vi "User Log In (popup).vi"(8 "error in (no error)":errorcluster, 11 "Path":path=path "R:/Freelancing/BEL/RMU LV Code_ver8.0/Data/credentials.txt") -> (0 "error out":errorcluster, 1 "selected account name":string, 2 "test sequence file name":string, 3 "Stop App?":bool, 5 "Name indicator":string caption="Name(min 4 chars)")   [LabVIEW 2021]
uses:
  controls/encryption.ctl
  <vilib>/event_ctls.llb/eventvkey.ctl
  <vilib>/Utility/file.llb/Write Delimited Spreadsheet (string).vi
  <vilib>/Utility/file.llb/Read Delimited Spreadsheet (string).vi
  <vilib>/regexp/Match Regular Expression.xnode
panel:
  in  "test sequence file":u16(ring) caption="Enum" items=["test sequence.seq", "test sequence1.seq", "vishal.seq"]
  out "Tab Control":enum32{"Login account", "Change Password"}(tab)
  in  "Account":enum16{"Administrator", "Operator"}(ring)
  in  "Password":string
  in  "Log In":bool
  out "Attempt":dbl
  out "Attempt (Max)":dbl
  out "lock/unlock":enum32{"lock", "unlock"}(tab)
  in  "Change Password":bool
  in  "Name":string caption="Name(min 4 chars)"
  in  "Account 2":enum16{"Administrator", "Operator"}(ring) caption="Account"
  in  "Password 2":string caption="Password"
  in  "New Password":string
  in  "Confirm Password":string
  in  "Update":bool
  in  "Home":bool
  out "selected account":enum16{"Administrator", "Operator"}(ring)
  # "Please select the appropriate user \naccount, enter the associated \npassword, then select Log In"
  # "Log In attempt"
  # "of"
  # "Please select the appropriate user \naccount, enter the new \npassword, then select Update"
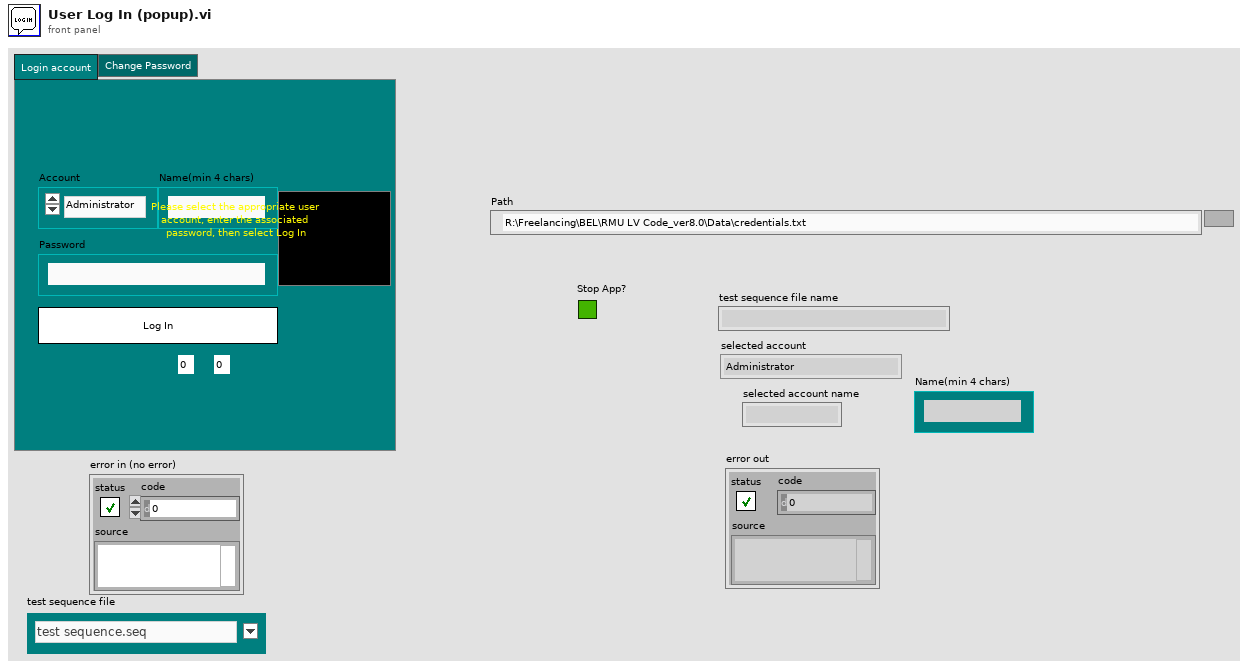
[diagram p1: front panel]
types:
  T1 = typedef "encryption.ctl" = enum16{"encode", "decode"}
  T2 = typedef "eventvkey.ctl" = enum16{"ASCII", "Enter", "Return", "Shift", "Ctrl", "Alt", "Cmd", "Opt", "Caps", "NumLock", "Clear", "Break", "Up", "Down", "Left", "Right", "Insert", "Delete", "Home", "End", "PageUp", "PageDown", "Escape", "Help", "Pause", "ScrollLock", "F1", "F2", "F3", "F4", "F5", "F6", "F7", "F8", "F9", "F10", "F11", "F12", "F13", "F14", "F15", "F16", "F17", "F18", "F19", "F20", "F21", "F22", "F23", "F24", "Play", "VolumeUp", "VolumeDown", "Mute", "Two Byte Char"}
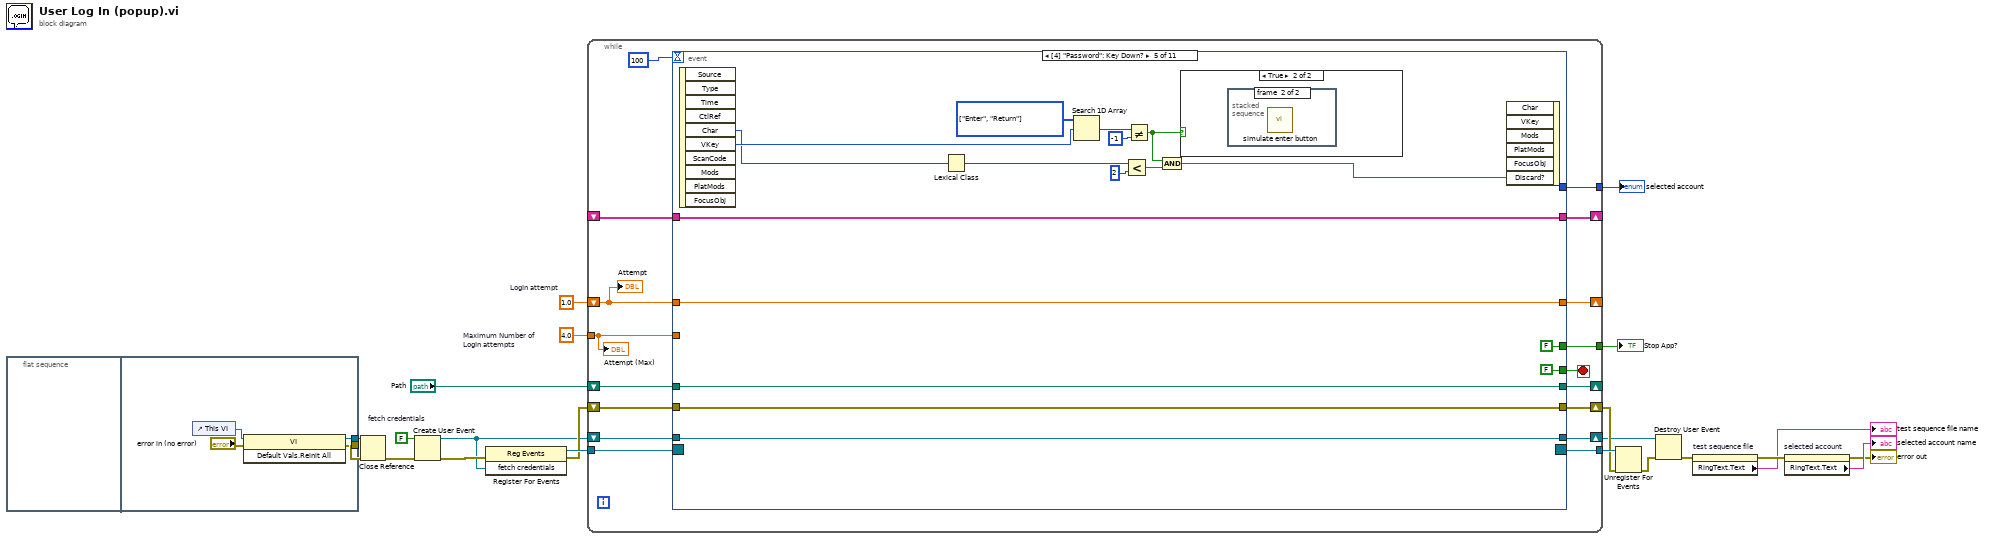
[diagram p0: block diagram]
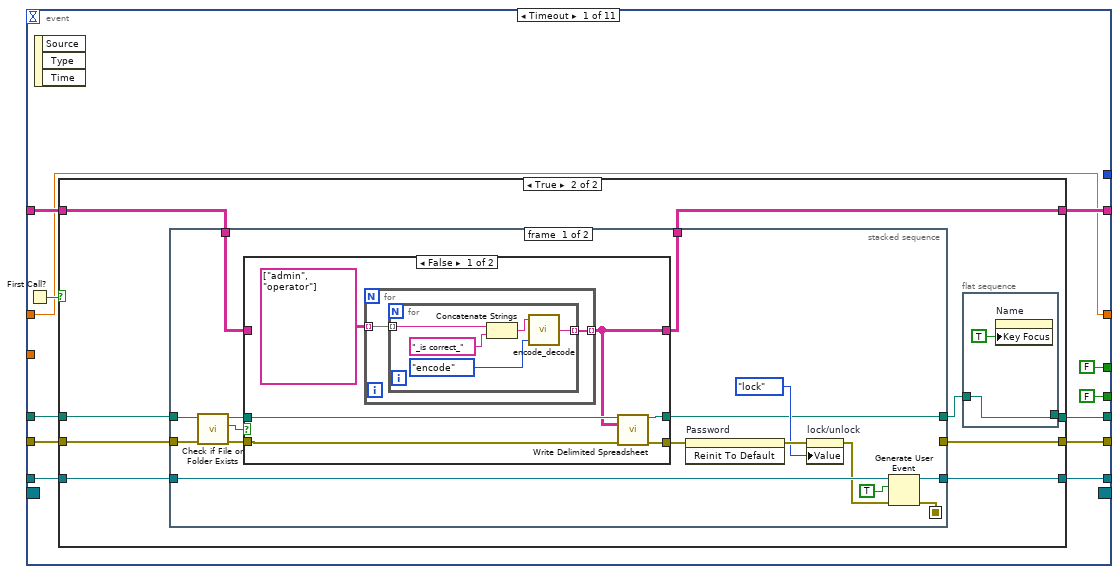
[diagram p2: hidden frame]
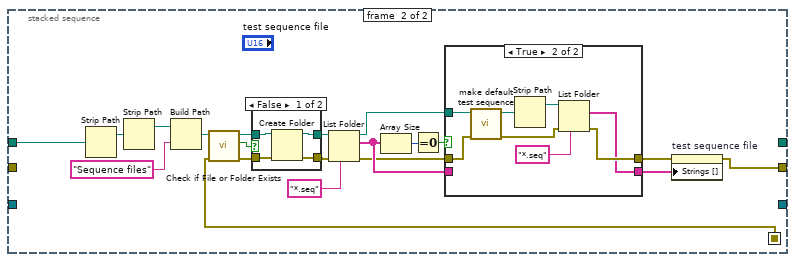
[diagram p5: hidden frame]
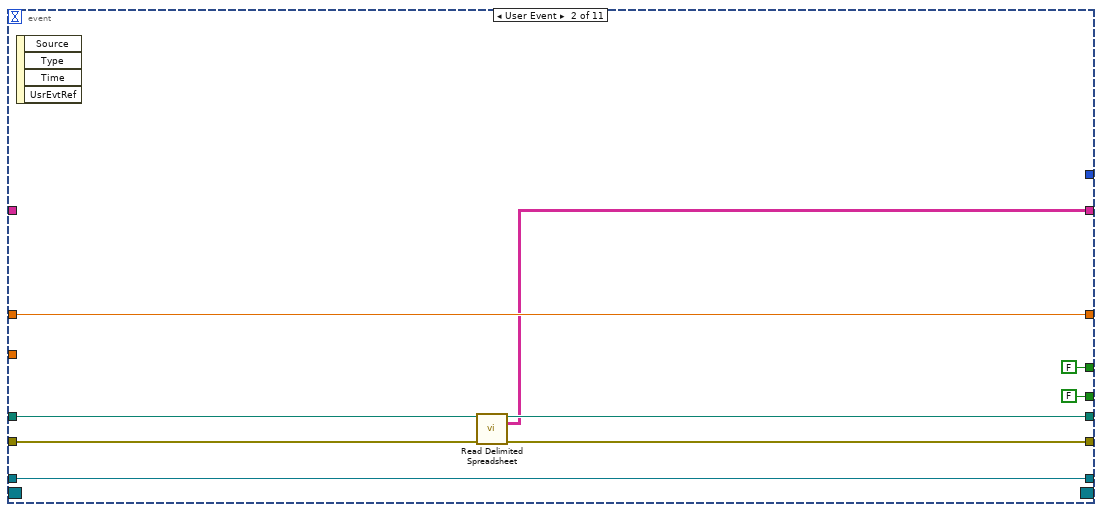
[diagram p8: hidden frame]
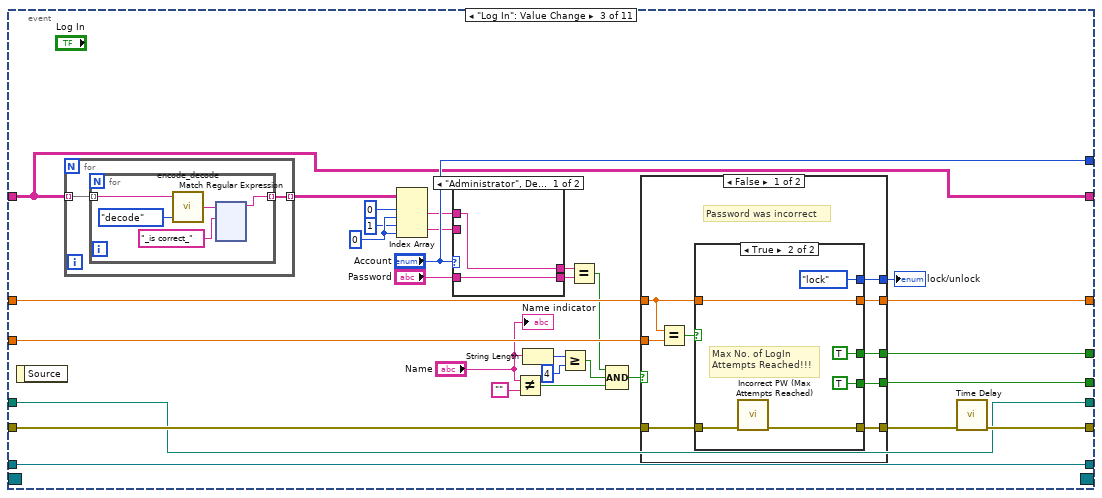
[diagram p9: hidden frame]
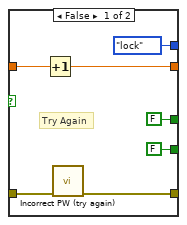
[diagram p10: hidden frame]
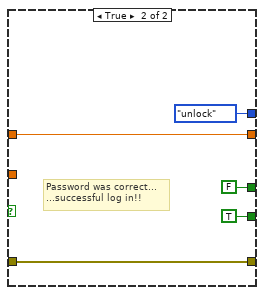
[diagram p11: hidden frame]
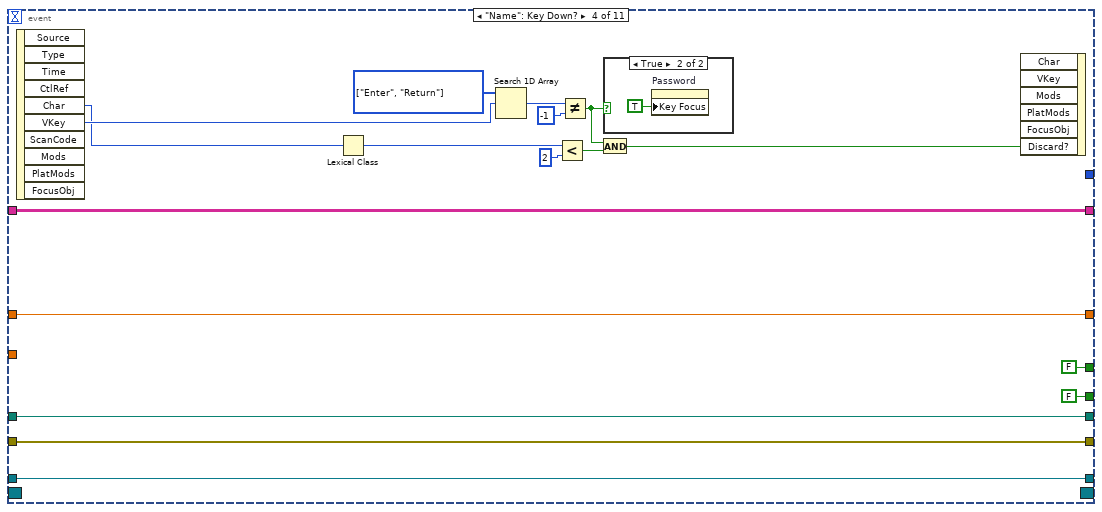
[diagram p13: hidden frame]
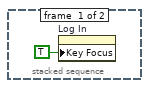
[diagram p16: hidden frame]
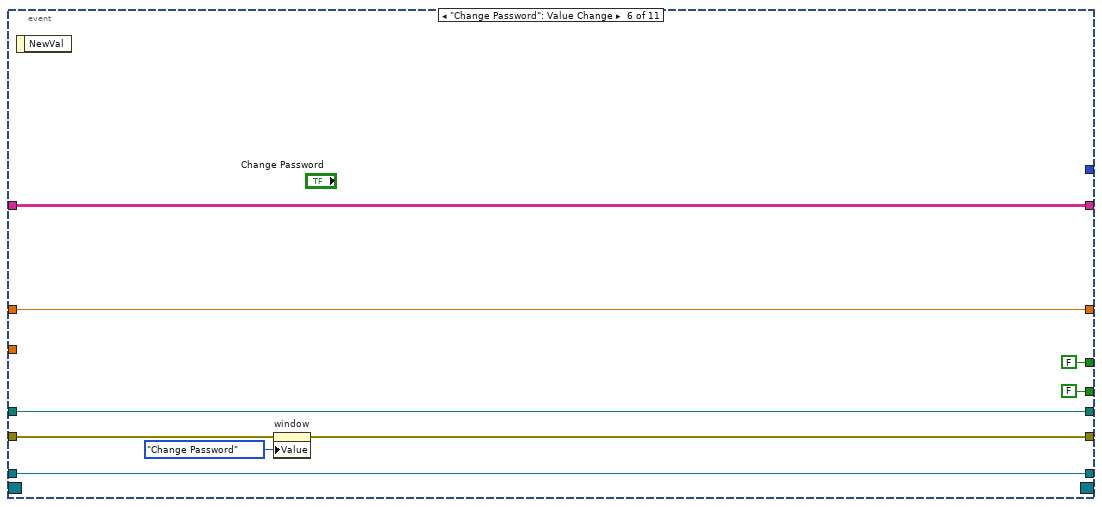
[diagram p17: hidden frame]
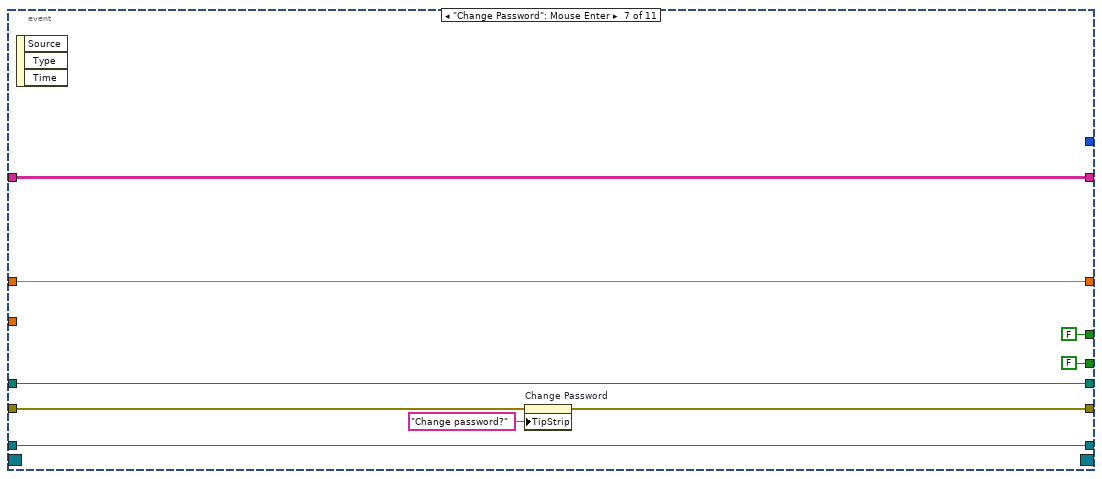
[diagram p18: hidden frame]
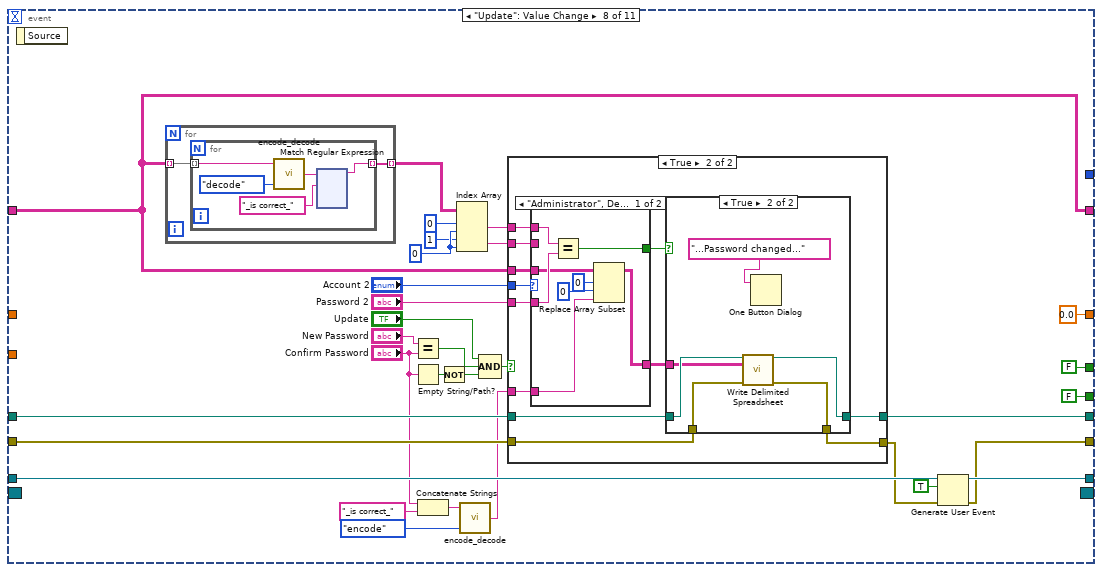
[diagram p19: hidden frame]
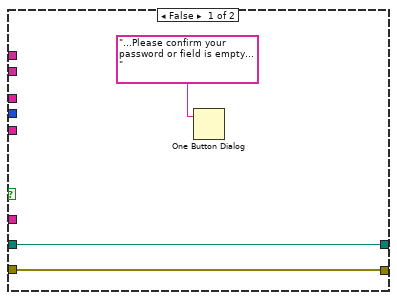
[diagram p20: hidden frame]
diagram:
  w18 = FALSE  # fetch credentials
  w21 = 1.0  # LogIn attempt
  w22 = 4.0  # Maximum Number of  LogIn attempts
  n1 = flat-sequence {
    tunnel: [w26] -> w9
    tunnel: [w23] -> w8
    frame #0 {
    }
    frame #1 {
      n2 = control-ref of="This VI"() -> (w25:refnum<vi>)
      n3 = invoke class="VI" method="Default Vals.Reinit All"(reference=w25, error in="error in (no error)") -> (reference out=w26:refnum<vi>, error out=w23:errorcluster)  [unwired: 1 in, 1 out]
    }
  }
  n4 = Close Reference(reference=w9, error in (no error)=w8) -> (error out=w7:errorcluster)
  n5 = Create User Event(user event datatype=w18, error in=w7) -> (user event=w14:refnum<user-event>, error out=w17:errorcluster)
  n6 = register-events(error in=w17, w14) -> (reference out=w16:refnum<event-registration>, error out=w15:errorcluster)  [unwired: 1 in]
  n7 = while {
    tunnel: w22 -> [w27]
    shift-right: [w42] -> _
    shift-left: w21 -> [w43]
    tunnel: [w40] -> w6
    tunnel: [w39] -> w19
    shift-right: [w34] -> _
    shift-left: "Path" -> [w37]
    shift-right: [w35] -> w12
    shift-left: w15 -> [w38]
    shift-right: [w33] -> _
    shift-left: _ -> [w32]
    tunnel: w16 -> [w31]
    shift-right: [w29] -> w11
    shift-left: w14 -> [w30]
    tunnel: [w28] -> w13
    stop <- w41 stop-if-true
    n8 = event shown="[4] \"Password\": Key Down?" {
      selector: w31 -> [_ _ _ _ _ _ _ _ _ _ _]
      dyn-events: [_ _ _ _ _ _ _ _ _ _ _] -> w28
      timeout: 100 -> [_ _ _ _ _ _ _ _ _ _ _]
      tunnel: w43 -> [w44 w144 w174 w338 w356 w370 w379 _ w583 w593 w605]
      tunnel: [w44 w144 w173 w338 w356 w370 w379 0.0 ("LogIn attempt") w583 w593 w605] -> w42
      tunnel: [FALSE FALSE w172 FALSE FALSE FALSE FALSE FALSE FALSE FALSE TRUE] -> w41
      tunnel: w27 -> [_ _ w171 _ _ _ _ _ _ _ _]
      tunnel: [FALSE FALSE w170 FALSE FALSE FALSE FALSE FALSE FALSE FALSE TRUE] -> w40
      tunnel: [_ _ "Account" _ _ _ _ _ _ _ _] -> w39
      tunnel: w38 -> [w54 w146 w168 w336 w354 w376 w386 w400 w588 w598 w602]
      tunnel: w37 -> [w55 w147 w159 w337 w355 w374 w383 w404 w587 w594 w603]
      tunnel: [w52 w145 w160 w336 w354 w375 w385 w395 w588 w597 w602] -> w35
      tunnel: [w53 w143 w159 w337 w355 w374 w383 w403 w587 w594 w603] -> w34
      tunnel: [w51 w142 w148 w339 w357 w371 w380 w388 w584 w595 w604] -> w33
      tunnel: w32 -> [w49 _ w148 w339 w357 w371 w380 w388 w584 w595 w604]
      tunnel: w30 -> [w45 w141 w157 w333 w351 w369 w378 w399 w582 w592 w601]
      tunnel: [w46 w141 w157 w333 w351 w369 w378 w398 w582 w592 w601] -> w29
      event Timeout {
        n9 = First Call?() -> (First Call?: T/F=w50:bool)
        n10 = event-data() -> ()  [unwired: 1 in, 3 out]
        n11 = case shown="True" w50 {
          tunnel: w55 -> [w58 w68]
          tunnel: w54 -> [w57 w67]
          tunnel: [w58 w61] -> w53
          tunnel: [w57 w62] -> w52
          tunnel: [w59 w64] -> w51
          tunnel: w49 -> [w59 w63]
          tunnel: [w56 w66] -> w46
          tunnel: w45 -> [w56 w65]
          frame False {
          }
          frame True {
            n12 = stacked-sequence {
              seq-local: [w71 _] -> [_ w110]
              tunnel: w68 -> [w80 w114]
              tunnel: w67 -> [w79 _]
              tunnel: [w78 _] -> w60
              tunnel: [w77 _] -> w66
              tunnel: w65 -> [w76 _]
              tunnel: [w73 _] -> w64
              tunnel: w63 -> [w72 _]
              tunnel: [_ w109] -> w62
              frame #0 {
                n13 = call <vilib>:"Check if File or Folder Exists.vi"("error in (no error)"=w79, "path"=w80) -> ("error out"=w84:errorcluster, "file or folder exists?"=w82:bool, "dup path"=w83:path)  [unwired: 7 in]
                n14 = case shown="False" w82 {
                  tunnel: w83 -> [w92 w102]
                  tunnel: w84 -> [w91 w101]
                  tunnel: [w90 w102] -> w78
                  tunnel: [w89 w101] -> w85
                  tunnel: [w87 w100] -> w73
                  tunnel: w72 -> [_ w100]
                  frame False {
                    n15 = for {
                      tunnel: string[][] [["admin"], ["operator"]] -> [w94] mode=indexing
                      tunnel: [w93] -> w87 mode=indexing
                      n16 = for {
                        tunnel: w94 -> [w99] mode=indexing
                        tunnel: [w96] -> w93 mode=indexing
                        n17 = Concatenate Strings(w99, "_is correct_") -> (w97:string)
                        n18 = call "encode_decode.vi"("Enum"=encryption."encode", "Input string"=w97) -> ("encoded/decoded string"=w96:string)  [unwired: 1 in]
                      }
                    }
                    n19 = call-poly <vilib>:"Write Delimited Spreadsheet.vi"("file path (dialog if empty)"=w92, "2D data"=w87, "error in (no error)"=w91) -> ("new file path (Not A Path if cancelled)"=w90:path, "error out"=w89:errorcluster)  [unwired: 11 in]
                  }
                  frame True {
                  }
                }
                n20 = invoke on="Password" class="Str" method="Reinit To Default"(error in=w85) -> (error out=w86:errorcluster)  [unwired: 2 in, 2 out]
                n21 = property on="lock/unlock" class="TabCtl (strict)"(error in=w86, "Value"=enum32{"lock", "unlock"}."lock" ("lock/unlock")) -> (error out=w74:errorcluster)  [unwired: 1 in, 1 out]
                n22 = Generate User Event(user event=w76, event data cluster=TRUE ("event data"), error in=w74) -> (user event out=w77:refnum<user-event>, error out=w71:errorcluster)  [unwired: 1 in]
              }
              frame #1 {
                n23 = Strip Path(path=w114) -> (stripped path=w116:path)  [unwired: 1 out]
                n24 = Strip Path(path=w116) -> (stripped path=w122:path)  [unwired: 1 out]
                n25 = Build Path(base path=w122, name or relative path="Sequence files") -> (appended path=w120:path)
                n26 = call <vilib>:"Check if File or Folder Exists.vi"("error in (no error)"=w110, "path"=w120) -> ("error out"=w117:errorcluster, "file or folder exists?"=w119:bool, "dup path"=w118:path)  [unwired: 7 in]
                n27 = case shown="False" w119 {
                  tunnel: w118 -> [w136 w138]
                  tunnel: w117 -> [w135 w137]
                  tunnel: [w134 w138] -> w115
                  tunnel: [w133 w137] -> w112
                  frame False {
                    n28 = Create Folder(path (use dialog)=w136, error in=w135) -> (created path=w134:path, error out=w133:errorcluster)  [unwired: 1 in, 1 out]
                  }
                  frame True {
                  }
                }
                n29 = List Folder(path=w115, pattern="*.seq", error in=w112) -> (path out=w105:path, filenames=w107:string[], error out=w104:errorcluster)  [unwired: 1 in, 1 out]
                n30 = Array Size(array=w107) -> (size(s)=w111:i32)
                n31 = Equal To 0?(x=w111) -> (x = 0?=w108:bool)
                n32 = case shown="True" w108 {
                  tunnel: w107 -> [w124 _]
                  tunnel: [w124 w125] -> w106
                  tunnel: w105 -> [_ w132]
                  tunnel: w104 -> [w123 w131]
                  tunnel: [w123 w126] -> w103
                  frame False {
                  }
                  frame True {
                    n33 = call "make default test sequence.vi"("error in"=w131, "file path"=w132) -> ("error out"=w127:errorcluster, "new file path"=w130:path)  [unwired: 8 in]
                    n34 = Strip Path(path=w130) -> (stripped path=w129:path)  [unwired: 1 out]
                    n35 = List Folder(path=w129, pattern="*.seq", error in=w127) -> (filenames=w125:string[], error out=w126:errorcluster)  [unwired: 1 in, 2 out]
                  }
                }
                n36 = property on="test sequence file" class="Ring (strict)"(error in=w103, "Strings []"=w106) -> (error out=w109:errorcluster)  [unwired: 1 in, 1 out]
              }
            }
            n37 = flat-sequence {
              tunnel: [w69] -> w61
              tunnel: w60 -> [w69]
              frame #0 {
                n38 = property on="Name" class="Str"("Key Focus"=TRUE) -> ()  [unwired: 2 in, 2 out]
              }
            }
          }
        }
      }
      event User Event {
        n39 = event-data() -> ()  [unwired: 1 in, 4 out]
        n40 = call-poly <vilib>:"Read Delimited Spreadsheet.vi"("file path (dialog if empty)"=w147, "error in (no error)"=w146) -> ("new file path (Not A Path if cancelled)"=w143:path, "all rows"=w142:string[][], "error out"=w145:errorcluster)  [unwired: 8 in, 3 out]
      }
      event "Log In": Value Change {
        w167 = 0 ("disabled index (col)")
        n41 = event-data() -> ()  [unwired: 1 in, 1 out]
        n42 = for {
          tunnel: w148 -> [w179] mode=indexing
          tunnel: [w178] -> w158 mode=indexing
          n43 = for {
            tunnel: w179 -> [w184] mode=indexing
            tunnel: [w180] -> w178 mode=indexing
            n44 = call "encode_decode.vi"("Enum"=encryption."decode", "Input string"=w184) -> ("encoded/decoded string"=w182:string)  [unwired: 1 in]
            n45 = xnode "Match Regular Expression"("input string"=w182, "regular expression"="_is correct_") -> ("before match"=w180:string)  [unwired: 4 in, 4 out]
          }
        }
        n46 = Index Array(array=w158, index (row) #1=0 ("disabled index (row)"), index (col) #1=w167, index (row) #2=1 ("disabled index (row)"), index (col) #2=w167) -> (element #1=w164:string, element #2=w163:string)
        n47 = case shown="\"Administrator\", Default" "Account" {
          tunnel: "Password" -> [w330 w332]
          tunnel: [w330 w332] -> w176
          tunnel: [w329 w331] -> w175
          tunnel: w164 -> [w329 _]
          tunnel: w163 -> [_ w331]
          frame "Administrator", Default {
          }
          frame "Operator" {
          }
        }
        n48 = Not Equal?(x="Name", y="") -> (x != y?=w151:bool)
        n49 = String Length(string="Name") -> (length=w154:i32)
        n50 = Greater Or Equal?(x=w154, y=4) -> (x >= y?=w152:bool)
        n51 = Equal?(x=w175, y=w176) -> (x = y?=w150:bool)
        n52 = Compound Arithmetic op=AND(w150, w152, w151) -> (w149:bool)
        n53 = case shown="False" w149 {
          tunnel: w174 -> [w308 w328]
          tunnel: [w307 w328] -> w173
          tunnel: [w305 TRUE] -> w172
          tunnel: w171 -> [w309 _]
          tunnel: [w306 FALSE] -> w170
          tunnel: w168 -> [w304 w325]
          tunnel: [w303 w325] -> w162
          tunnel: [w302 enum32{"lock", "unlock"}."unlock" ("lock/unlock")] -> w161
          frame False {
            # "Password was incorrect"
            n54 = Equal?(x=w308, y=w309) -> (x = y?=w310:bool)
            n55 = case shown="True" w310 {
              tunnel: w308 -> [w317 w323]
              tunnel: [w316 w323] -> w307
              tunnel: [FALSE TRUE] -> w306
              tunnel: [FALSE TRUE] -> w305
              tunnel: w304 -> [w313 w320]
              tunnel: [w312 w319] -> w303
              tunnel: [enum32{"lock", "unlock"}."lock" ("lock/unlock") enum32{"lock", "unlock"}."lock" ("lock/unlock")] -> w302
              frame False {
                # "Try Again"
                n56 = Increment(x=w317) -> (x+1=w316:dbl)
                n57 = call "Incorrect PW (try again).vi"("error in (no error)"=w313) -> ("error out"=w312:errorcluster)  [unwired: 10 in]
              }
              frame True {
                # "Max No. of LogIn\nAttempts Reached!!!"
                n58 = call "Incorrect PW (Max Attempts Reached).vi"("error in (no error)"=w320) -> ("error out"=w319:errorcluster)  [unwired: 10 in]
              }
            }
          }
          frame True {
            # "Password was correct...\n...successful log in!!"
          }
        }
        "lock/unlock" <- w161
        n59 = call "Time Delay"("error in (no error)"=w162) -> ("error out"=w160:errorcluster)  [unwired: 10 in]
        "Name indicator" <- "Name"
      }
      event "Name": Key Down? {
        w349 = T2[] [enum."Enter", enum."Return"] items=["ASCII", "Enter", "Return", "Shift", "Ctrl", "Alt", "Cmd", "Opt", "Caps", "NumLock", "Clear", "Break", "Up", "Down", "Left", "Right", "Insert", "Delete", "Home", "End", "PageUp", "PageDown", "Escape", "Help", "Pause", "ScrollLock", "F1", "F2", "F3", "F4", "F5", "F6", "F7", "F8", "F9", "F10", "F11", "F12", "F13", "F14", "F15", "F16", "F17", "F18", "F19", "F20", "F21", "F22", "F23", "F24", "Play", "VolumeUp", "VolumeDown", "Mute", "Two Byte Char"]
        n60 = event-data() -> ("Char"=w342:i16, "VKey"=w343:T2)  [unwired: 1 in, 8 out]
        n61 = Lexical Class(1:w342) -> (0:w348:i16)
        n62 = Search 1D Array(1D array=w349, element=w343) -> (index of element=w345:i32)  [unwired: 1 in]
        n63 = Less?(x=w348, y=i16 2) -> (x < y?=w346:bool)
        n64 = Not Equal?(x=w345, y=-1) -> (x != y?=w340:bool)
        n65 = And(x=w340, y=w346) -> (x .and. y?=w341:bool)
        n66 = case shown="True" w340 {
          frame False {
          }
          frame True {
            n67 = property on="Password" class="Str"("Key Focus"=TRUE) -> ()  [unwired: 2 in, 2 out]
          }
        }
        n68 = event-data("Discard?"=w341) -> ()  [unwired: 6 in, 1 out]
      }
      event "Password": Key Down? {
        w367 = T2[] [enum."Enter", enum."Return"] items=["ASCII", "Enter", "Return", "Shift", "Ctrl", "Alt", "Cmd", "Opt", "Caps", "NumLock", "Clear", "Break", "Up", "Down", "Left", "Right", "Insert", "Delete", "Home", "End", "PageUp", "PageDown", "Escape", "Help", "Pause", "ScrollLock", "F1", "F2", "F3", "F4", "F5", "F6", "F7", "F8", "F9", "F10", "F11", "F12", "F13", "F14", "F15", "F16", "F17", "F18", "F19", "F20", "F21", "F22", "F23", "F24", "Play", "VolumeUp", "VolumeDown", "Mute", "Two Byte Char"]
        n69 = event-data() -> ("Char"=w360:i16, "VKey"=w361:T2)  [unwired: 1 in, 8 out]
        n70 = Lexical Class(1:w360) -> (0:w366:i16)
        n71 = Search 1D Array(1D array=w367, element=w361) -> (index of element=w363:i32)  [unwired: 1 in]
        n72 = Less?(x=w366, y=i16 2) -> (x < y?=w364:bool)
        n73 = Not Equal?(x=w363, y=-1) -> (x != y?=w358:bool)
        n74 = And(x=w358, y=w364) -> (x .and. y?=w359:bool)
        n75 = case shown="True" w358 {
          frame False {
          }
          frame True {
            n76 = stacked-sequence {
              frame #0 {
                n77 = property on="Log In" class="Bool (strict)"("Key Focus"=TRUE) -> ()  [unwired: 2 in, 2 out]
              }
              frame #1 {
                n78 = call "simulate enter button.vi"() -> ()  [unwired: 12 in]
              }
            }
          }
        }
        n79 = event-data("Discard?"=w359) -> ()  [unwired: 6 in, 1 out]
      }
      event "Change Password": Value Change {
        n80 = event-data() -> ()  [unwired: 1 in, 1 out]
        n81 = property on="window" class="TabCtl (strict)"(error in=w376, "Value"=enum32{"Login account", "Change Password"}."Change Password" ("Tab Control")) -> (error out=w375:errorcluster)  [unwired: 1 in, 1 out]
      }
      event "Change Password": Mouse Enter {
        n82 = event-data() -> ()  [unwired: 1 in, 3 out]
        n83 = property on="Change Password" class="Bool"(error in=w386, "TipStrip"="Change password?" ("Tip Strip")) -> (error out=w385:errorcluster)  [unwired: 1 in, 1 out]
      }
      event "Update": Value Change {
        w409 = 0 ("disabled index (col)")
        n84 = event-data() -> ()  [unwired: 1 in, 1 out]
        n85 = for {
          tunnel: w388 -> [w419] mode=indexing
          tunnel: [w418] -> w387 mode=indexing
          n86 = for {
            tunnel: w419 -> [w424] mode=indexing
            tunnel: [w420] -> w418 mode=indexing
            n87 = call "encode_decode.vi"("Enum"=encryption."decode", "Input string"=w424) -> ("encoded/decoded string"=w422:string)  [unwired: 1 in]
            n88 = xnode "Match Regular Expression"("input string"=w422, "regular expression"="_is correct_") -> ("before match"=w420:string)  [unwired: 4 in, 4 out]
          }
        }
        n89 = Equal?(x="New Password", y="Confirm Password") -> (x = y?=w413:bool)
        n90 = Empty String/Path?(string/path="Confirm Password") -> (empty?=w416:bool)
        n91 = Concatenate Strings("Confirm Password", "_is correct_") -> (w393:string)
        n92 = Not(x=w416) -> (.not. x?=w415:bool)
        n93 = Index Array(array=w387, index (row) #1=0 ("disabled index (row)"), index (col) #1=w409, index (row) #2=1 ("disabled index (row)"), index (col) #2=w409) -> (element #1=w407:string, element #2=w406:string)
        n94 = call "encode_decode.vi"("Enum"=encryption."encode", "Input string"=w393) -> ("encoded/decoded string"=w389:string)  [unwired: 1 in]
        n95 = Compound Arithmetic op=AND("Update", w413, w415) -> (w417:bool)
        n96 = case shown="True" w417 {
          tunnel: "Account 2" -> [_ w556]
          tunnel: w407 -> [_ w555]
          tunnel: w406 -> [_ w554]
          tunnel: "Password 2" -> [_ w553]
          tunnel: w388 -> [_ w552]
          tunnel: w389 -> [_ w551]
          tunnel: w404 -> [w543 w549]
          tunnel: w400 -> [w544 w547]
          tunnel: [w544 w546] -> w396
          tunnel: [w543 w545] -> w403
          frame False {
            n97 = One Button Dialog(message="...Please confirm your password or field is empty...") -> ()  [unwired: 1 in, 1 out]
          }
          frame True {
            n98 = case shown="\"Administrator\", Default" w556 {
              tunnel: w555 -> [w573 _]
              tunnel: w554 -> [_ w576]
              tunnel: w553 -> [w572 w581]
              tunnel: w552 -> [w571 w580]
              tunnel: w551 -> [w568 w577]
              tunnel: [w567 w575] -> w550
              tunnel: [w566 w574] -> w548
              frame "Administrator", Default {
                n99 = Equal?(x=w573, y=w572) -> (x = y?=w567:bool)
                n100 = Replace Array Subset(array=w571, new element=w568, index (row)=0, index (col)=0 ("disabled index (col)")) -> (w566:string[][])
              }
              frame "Operator" {
                n101 = Equal?(x=w576, y=w581) -> (x = y?=w575:bool)
                n102 = Replace Array Subset(array=w580, new element=w577, index (row)=0, index (col)=1 ("disabled index (col)")) -> (w574:string[][])
              }
            }
            n103 = case shown="True" w550 {
              tunnel: w549 -> [w557 w564]
              tunnel: w548 -> [_ w563]
              tunnel: w547 -> [w558 w562]
              tunnel: [w558 w561] -> w546
              tunnel: [w557 w560] -> w545
              frame False {
                n104 = One Button Dialog(message="...Incorrect old password...") -> ()  [unwired: 1 in, 1 out]
              }
              frame True {
                n105 = call-poly <vilib>:"Write Delimited Spreadsheet.vi"("file path (dialog if empty)"=w564, "2D data"=w563, "error in (no error)"=w562) -> ("new file path (Not A Path if cancelled)"=w560:path, "error out"=w561:errorcluster)  [unwired: 11 in]
                n106 = One Button Dialog(message="...Password changed...") -> ()  [unwired: 1 in, 1 out]
              }
            }
          }
        }
        n107 = Generate User Event(user event=w399, event data cluster=TRUE ("event data"), error in=w396) -> (user event out=w398:refnum<user-event>, error out=w395:errorcluster)  [unwired: 1 in]
      }
      event "Home": Value Change {
        n108 = event-data() -> ()  [unwired: 1 in, 6 out]
        "Tab Control" <- enum32{"Login account", "Change Password"}."Login account" ("Tab Control")
      }
      event "Home": Mouse Enter {
        n109 = event-data() -> ()  [unwired: 1 in, 4 out]
        n110 = property on="Home" class="Bool"(error in=w598, "TipStrip"="Home: go to login window?" ("Tip Strip")) -> (error out=w597:errorcluster)  [unwired: 1 in, 1 out]
      }
      event Panel Close? {
        n111 = event-data() -> ()  [unwired: 1 in, 4 out]
        n112 = event-data("Discard?"=TRUE) -> ()  [unwired: 1 in, 1 out]
      }
    }
    "Attempt" <- w43
    "Attempt (Max)" <- w27
  }
  "Stop App?" <- w6
  "selected account" <- w19
  n113 = Unregister For Events(event registration refnum=w13, error in=w12) -> (error out=w10:errorcluster)
  n114 = Destroy User Event(user event=w11, error in=w10) -> (error out=w5:errorcluster)
  n115 = property on="test sequence file" class="Ring (strict)"(error in=w5) -> (error out=w3:errorcluster, "RingText.Text"=→"test sequence file name":string)  [unwired: 1 in, 1 out]
  n116 = property on="selected account" class="Enum (strict)"(error in=w3) -> (error out=→"error out":errorcluster, "RingText.Text"=→"selected account name":string)  [unwired: 1 in, 1 out]
